vi "delete-from-data-table-by-tag.vi"(7 "frame.tag":string, 8 "error in (no error)":errorcluster, 11 "CANtable in":refnum<class "bAPPdata.lvclass">) -> (0 "error out":errorcluster, 3 "CANtable out":refnum<class "bAPPdata.lvclass">)   [LabVIEW 2015, in "bAPPdata.lvclass"]
uses:
  bAPPdata.lvclass
  bAPPdata.lvclass/bAPPdata.ctl
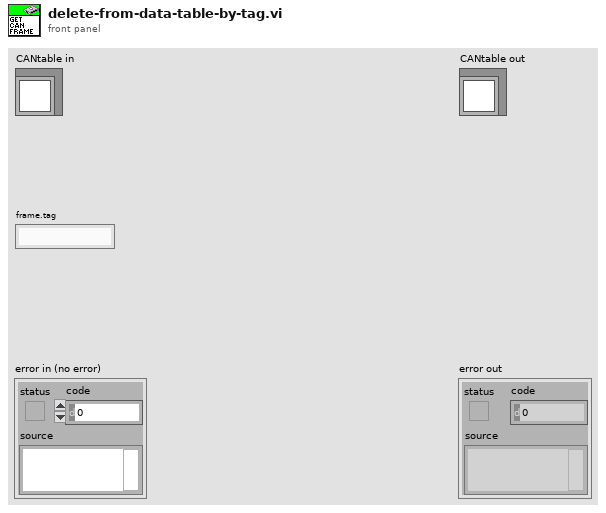
[diagram p1: front panel]
types:
  T1 = typedef "bAPPdata.lvclass/table-data.ctl" = T2[]
  T2 = typedef "bAPPdata.lvclass/table-contents.ctl" = cluster{"id":u32, "tag":string, "frame.type":T3, "last.frame":T4, "tMsgData":T6, "child.tags":string[], "bit-payload":bool[]}
  T3 = typedef "frame.type.ctl" = enum16{"FRAME NOT DEFINED", "DUT OUTPUT FRAME", "DUT INPUT FRAME"}
  T4 = typedef "XNET Frame CAN.ctl" = cluster{"timestamp":timestamp, "payload":u8[], "identifier":u32, "type":T5, "extended?":bool, "echo?":bool}
  T5 = typedef "XNET Frame Type CAN.ctl" = u8
  T6 = typedef "nMsgData.ctl" = cluster{"dwID":u32, "count":u32, "dwCycleTime":dbl, "dwTime":dbl, "new msg":bool}
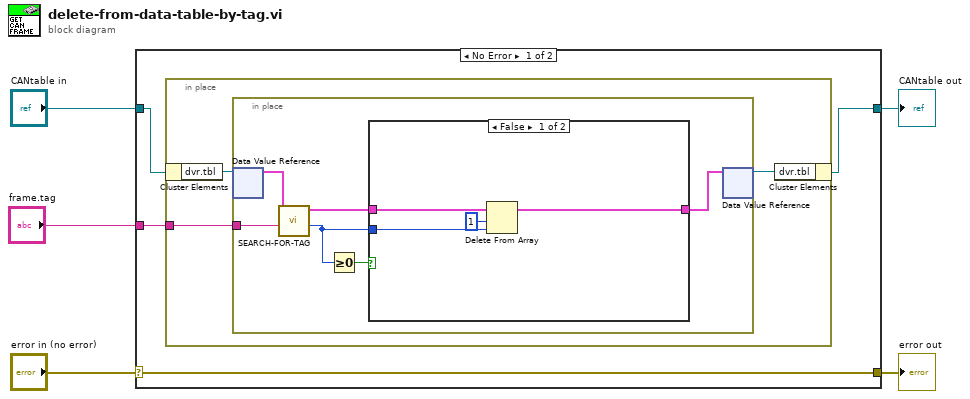
[diagram p0: block diagram]
diagram:
  n1 = case shown="No Error" "error in (no error)" {
    selector: "error in (no error)" -> [w9 w25]
    tunnel: [w9 w25] -> w4
    tunnel: [w7 w24] -> w2
    tunnel: "CANtable in" -> [w8 w24]
    tunnel: "frame.tag" -> [w6 _]
    frame No Error {
      n2 = in-place {
        in-place-border: w6 -> [w10]
        n3 = in-place-cluster #1(w8) -> ("dvr.tbl"=w12:refnum<data-value>)
        n4 = in-place {
          in-place-border: w10 -> [w17]
          n5 = in-place-dvr #2(w12) -> (w18:T1)  [unwired: 1 out]
          n6 = call "SEARCH-FOR-TAG.vi"("tag"=w17, "tbl.list"=w18) -> ("idx"=w13:i32, "tbl.list out"=w15:T2[])  [unwired: 8 in]
          n7 = Greater Or Equal To 0?(x=w13) -> (x >= 0?=w16:bool)
          n8 = case shown="False" w16 {
            tunnel: w15 -> [w22 w23]
            tunnel: [w21 w23] -> w14
            tunnel: w13 -> [w20 _]
            frame False {
              n9 = Delete From Array(array=w22, length=1, index=w20) -> (array with subset deleted=w21:T2[])  [unwired: 1 out]
            }
            frame True {
            }
          }
          n10 = in-place-dvr #2(w14) -> (w11:refnum<data-value>)  [unwired: 1 out]
        }
        n11 = in-place-cluster #1("dvr.tbl"=w11) -> (w7:refnum<class "bAPPdata.lvclass">)
      }
    }
    frame Error {
    }
  }
  "error out" <- w4
  "CANtable out" <- w2
